vi "Sound sample.vi"(10 "Sound  Input":path) -> (1 "Y":dbl[](array[numeric]), 2 "sound format":T1={"sample rate (S/s)"=22050.0, "number of channels"=2, "bits per sample"=16}, 3 "size(s)":i32)   [LabVIEW 2017]
uses:
  <vilib>/sound2/lvsound2.llb/Sound Data Format.ctl
  <vilib>/sound2/lvsound2.llb/Sound File Info (path).vi
  <vilib>/Utility/file.llb/Write Delimited Spreadsheet (DBL).vi
panel:
  out "Waveform Graph":waveform(dbl)(graph)
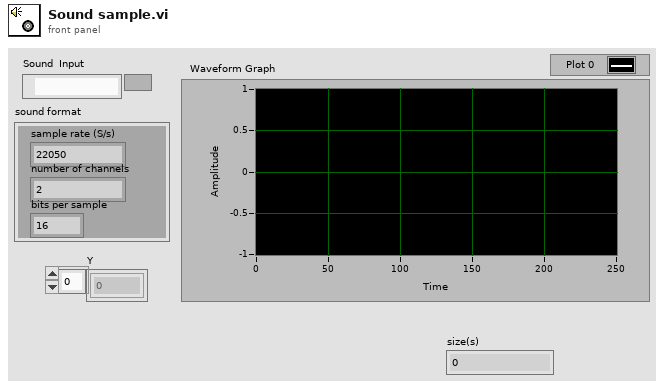
[diagram p1: front panel]
types:
  T1 = typedef "Sound Data Format.ctl" = cluster{"sample rate (S/s)":dbl, "number of channels":i32, "bits per sample":i32}
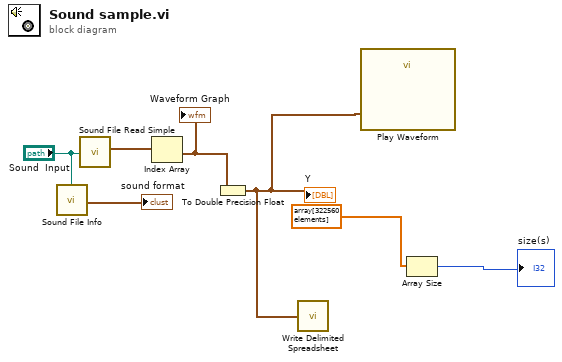
[diagram p0: block diagram]
diagram:
  n1 = call-poly <vilib>:"Sound File Info.vi"("path"="Sound  Input") -> ("sound format"=→"sound format":T1)  [unwired: 7 in, 3 out]
  n2 = call <vilib>:"Sound File Read Simple.vi"("path"="Sound  Input") -> ("data"=w5:waveform(dbl)[])  [unwired: 7 in, 3 out]
  n3 = Index Array(array=w5) -> (element=w4:waveform(dbl))  [unwired: 1 in]
  "Waveform Graph" <- w4
  n4 = To Double Precision Float(number=w4) -> (double precision float=w1:waveform(dbl))
  "Y" <- w1
  n5 = call-poly <vilib>:"Write Delimited Spreadsheet.vi"("1D data"=w1) -> ()  [unwired: 13 in, 2 out]
  n6 = call "Play Waveform"("Data"=w1) -> ()  [unwired: 18 in, 1 out]
  n7 = Array Size(array=dbl[] array[322560 elements] ("Y")) -> (size(s)=→"size(s)":i32)
